vi "EnergyContainer.vi"(4 "Capacity (FE)":ext, 5 "Last Fill (FE)":ext, 8 "Transfer (FE)":ext) -> (0 "Fill (FE)":ext, 1 "Needed (FE)":ext, 2 "Overflow":bool, 3 "Overflow (FE)":ext)   [LabVIEW 2026]
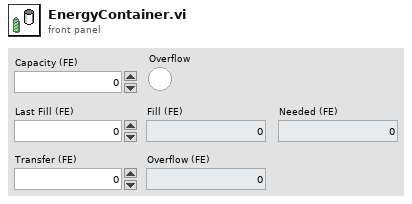
[diagram p1: front panel]
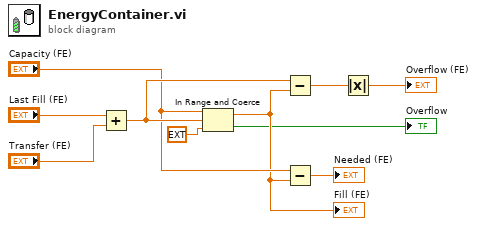
[diagram p0: block diagram]
diagram:
  n1 = Add(x="Last Fill (FE)", y="Transfer (FE)") -> (x+y=w7:ext)
  n2 = In Range and Coerce(upper limit="Capacity (FE)", x=w7, lower limit=ext 0.0) -> (coerced(x)=w4:ext, In Range?=→"Overflow":bool)
  "Fill (FE)" <- w4
  n3 = Subtract(x=w7, y=w4) -> (x-y=w6:ext)
  n4 = Subtract(x="Capacity (FE)", y=w4) -> (x-y=→"Needed (FE)":ext)
  n5 = Absolute Value(x=w6) -> (abs(x)=→"Overflow (FE)":ext)
